vi "PID_set_ratio.vi"() -> ()   [LabVIEW 2016]
uses:
  <vilib>/addons/control/pid/autopid.llb/PID autotuning parameters (adv).ctl
  <vilib>/Analysis/baseanly.llb/Mean (DBL).vi
  <userlib>/Fluigent/Fluigent MFCS/FluigentMFCS_Full.llb/MFCS_EZ Detect.vi
  <userlib>/Fluigent/Fluigent MFCS/FluigentMFCS_Full.llb/MFCS_EZ Initialization.vi
  <userlib>/Fluigent/Fluigent MFCS/FluigentMFCS_Full.llb/MFCS_EZ Read All Channels Pressure.vi
  <userlib>/Fluigent/Fluigent MFCS/FluigentMFCS_Full.llb/MFCS_EZ Write Channel Pressure.vi
  <vilib>/addons/control/pid/NI_PID_autopid.lvlib
  <vilib>/Analysis/NI_AALBase.lvlib
  <vilib>/addons/control/pid/autopid.llb/PID Autotuning Design (Auto).vi
panel:
  out "F0 Stable":dbl=817.2839885789583 format="%0.2f"
  out "Fw Stable":dbl=490.71052053591 format="%0.2f"
  out "F1 Stable":dbl=326.5734680430485 format="%0.2f"
  in  "Stable?":bool=TRUE
  out "Measured Ratio":dbl[](graph)
  out "Flow Setpoint":dbl=326.3448275862069
  in  "Ratio Setpoint":dbl=0.4
  in  "Set PID Gains":T1={"proportional gain (Kc)"=0.5, "integral time (Ti, min)"=0.03, "derivative time (Td, min)"=0.0} {"derivative time (Td, min)" format="%#.6g"; "integral time (Ti, min)" format="%#.6g"; "proportional gain (Kc)" format="%#.6g"}
  in  "Channels":enum16{"1", "2", "3", "4", "5", "6", "7", "8"}[](array[ring])=[enum."5", enum."6", enum."8"]
  in  "Boards":enum16{"A", "B", "C"}[](array[ring])=[enum."A", enum."A", enum."A"]
  out "error out":errorcluster
  out "dt":dbl=0.023001670837402344
  in  "Filter Size":i32=5
  out "Filtered Flow":dbl=326.84827586206893 format="%0.2f"
  out "Feedback Signal":dbl[](graph)
  out "Current F1":dbl=325.82758620689657
  out "tuning completed?":bool
  in  "Accept new parameters":bool
  out "tuned PID gains":T1={"proportional gain (Kc)"=0.5, "integral time (Ti, min)"=0.03, "derivative time (Td, min)"=0.0} {"derivative time (Td, min)" format="%#.6g"; "integral time (Ti, min)" format="%#.6g"; "proportional gain (Kc)" format="%#.6g"}
  in  "auto? (F)":bool=TRUE
  in  "autotuning parameters":T2={"technique"=1, "type of controller"=1, "control specification"=0, "amplitude"=10.0} {"amplitude" format="%.2f"; "control specification" items=["normal", "fast", "slow"]; "type of controller" items=["P", "PI", "PID"]; "technique" items=["Step Open Loop", "Step Closed Loop", "Relay", "PID Relay"]}
  in  "reinitialize? (F)":bool=TRUE
  in  "autotune? (F)":bool
  in  "Manual Pressure Set":dbl=300.0
  in  "Feedback on":bool=TRUE
  out "Flow Rate":dbl[](graph)
  out "Pressure":dbl[](graph)
  in  "stop":bool
  out "Pressure":dbl=554.8080444335938
  out "Feedback Signal":dbl=-0.25172413793100645 format="%.2f"
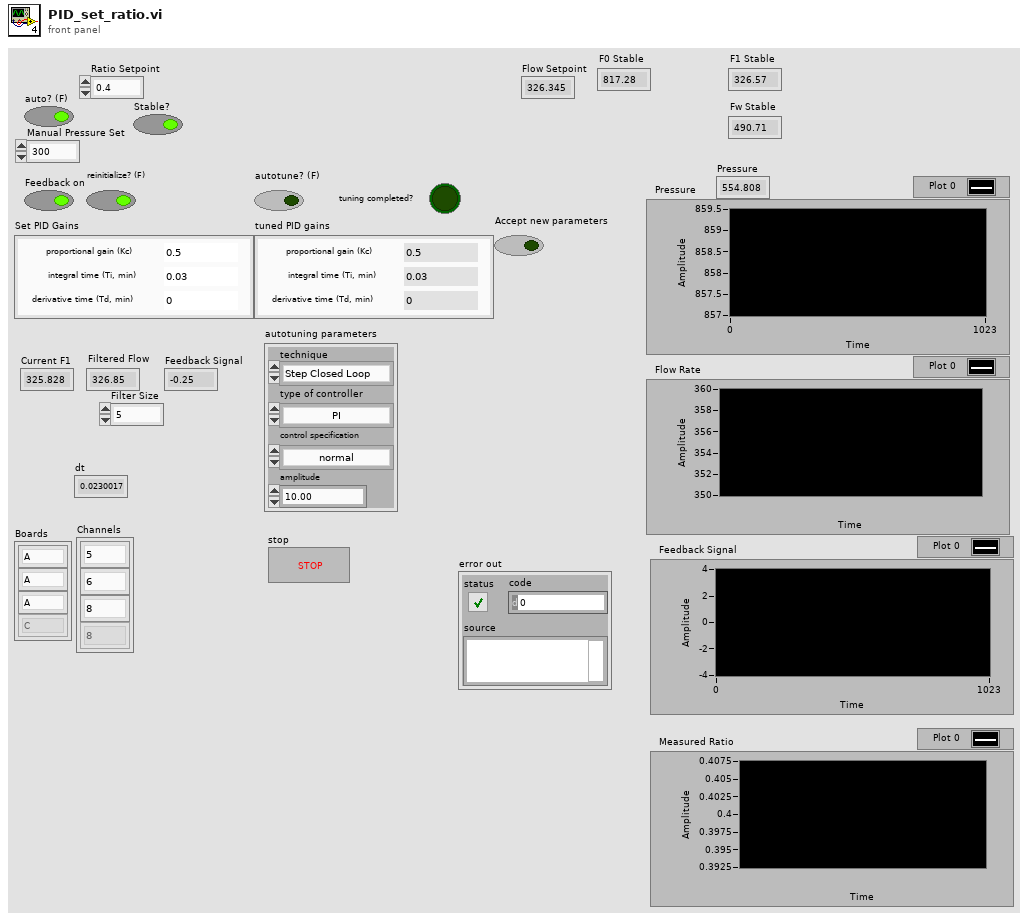
[diagram p1: front panel]
types:
  T1 = cluster{"proportional gain (Kc)":dbl, "integral time (Ti, min)":dbl, "derivative time (Td, min)":dbl}
  T2 = typedef "NI_PID_autopid.lvlib/PID autotuning parameters (adv).ctl" = cluster{"technique":u16, "type of controller":u16, "control specification":u16, "amplitude":dbl}
  T3 = typedef "_EZmfcsSN.ctl" = u16
  T4 = typedef "_frpRefNum" = refnum<k1>
  T5 = typedef "_EZmfcsRefNum.ctl" = refnum<k1>
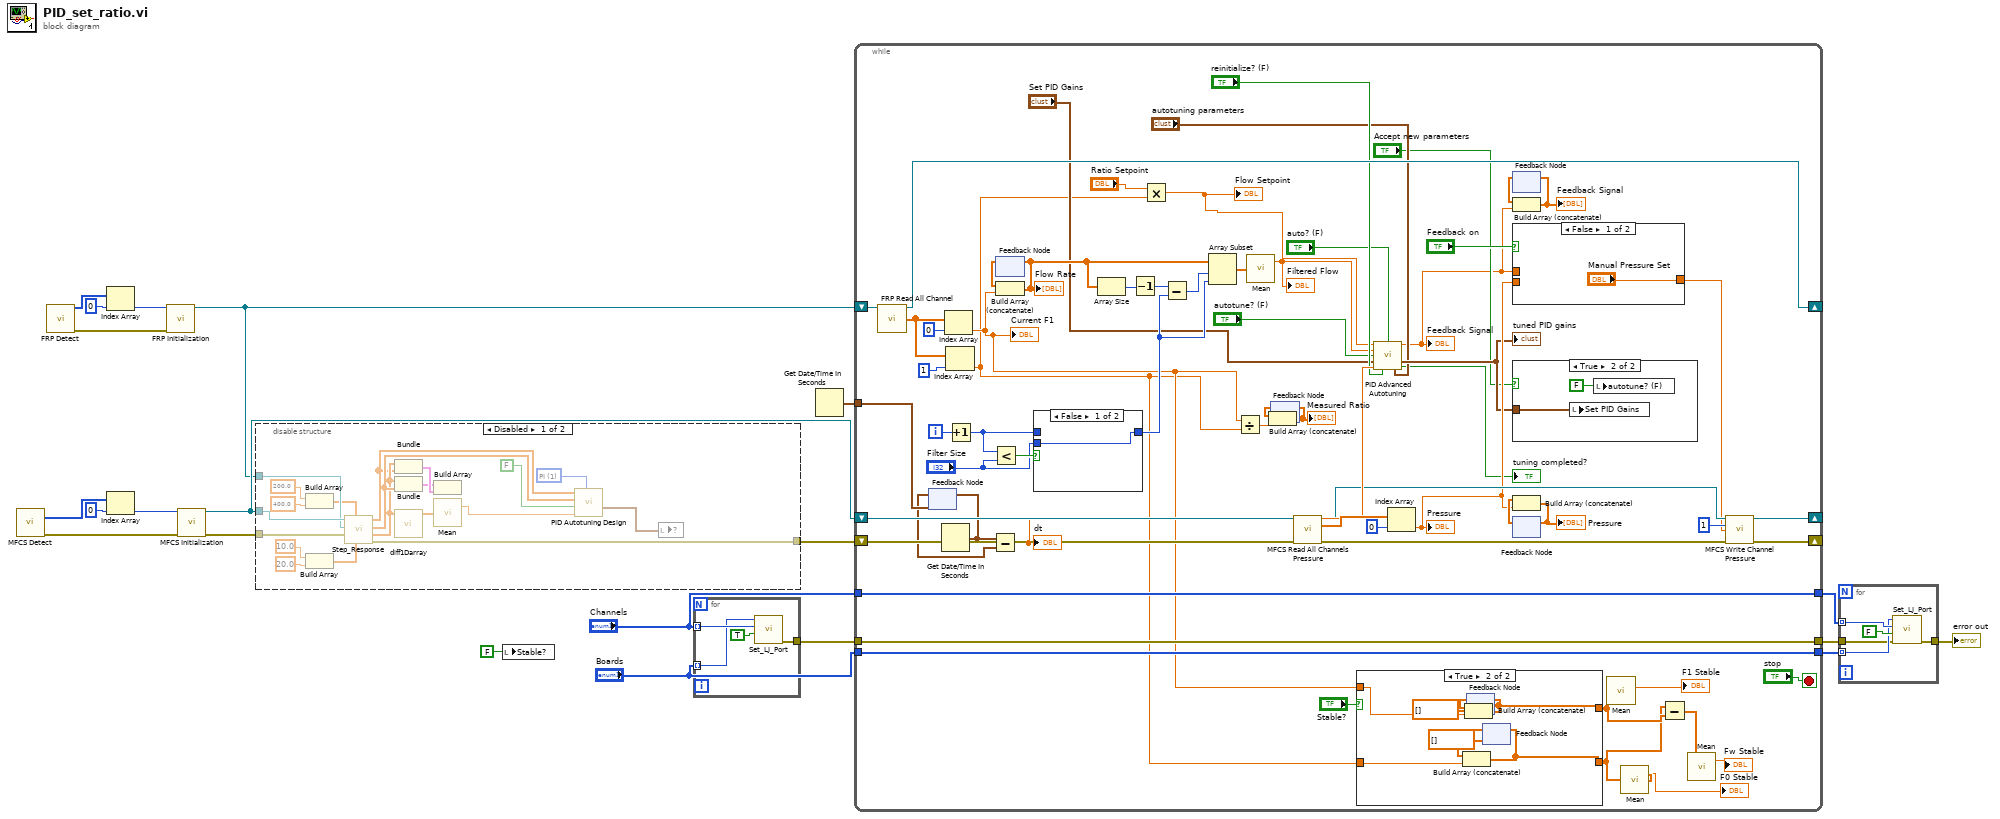
[diagram p0: block diagram]
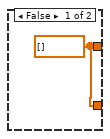
[diagram p3: hidden frame]
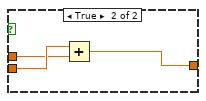
[diagram p6: hidden frame]
diagram:
  n1 = call-poly <userlib>:"MFCS Detect.vi"() -> ("[SN MFCS_EZ]"=w21:T3[], "error out"=w19:errorcluster)  [unwired: 14 in]
  n2 = call <userlib>:"FRP Detect.vi"() -> ("FLOWBOARD List"=w18:u16[], "error out"=w15:errorcluster)  [unwired: 14 in]
  n3 = Index Array(array=w18, index=0) -> (element=w14:u16)
  n4 = Index Array(array=w21, index=0) -> (element=w20:T3)
  n5 = call <userlib>:"FRP Initialization.vi"("Serial Number"=w14, "error in (no error)"=w15) -> ("FRP out"=w12:T4)  [unwired: 11 in, 2 out]
  n6 = call-poly <userlib>:"MFCS Initialization.vi"("SN MFCS_EZ"=w20, "error in (no error)"=w19) -> ("MFCS_EZ"=w13:T5, "error out"=w10:errorcluster)  [unwired: 11 in, 1 out]
  n7 = disable-structure shown="Disabled" {
    disable-tunnel: w13 -> [w43 _]
    disable-tunnel: w12 -> [w42 _]
    disable-tunnel: [w34 w44] -> w11
    disable-tunnel: w10 -> [w33 w44]
    frame Disabled {
      w38 = u16 1 items=["P", "PI", "PID"] ("Type of Controller")
      n8 = Build Array(200.0 ("element"), 400.0 ("element")) -> (w26:dbl[])
      n9 = Build Array(10.0 ("element"), 20.0 ("element")) -> (w27:dbl[])
      n10 = call "Step_Response.vi"("Times"=w27, "Pressure Sets"=w26, "MFCS Error"=w33, "FRP Handle"=w42, "MFCS Handle"=w43) -> ("error out"=w34:errorcluster, "T"=w25:dbl[], "Flow Rate"=w28:dbl[], "Pressure Setpoint"=w24:dbl[])  [unwired: 3 in]
      n11 = Bundle("T"=w25, "Pressure Setpoint"=w24) -> (w23:cluster{"T":dbl[], "Pressure Setpoint":dbl[]})  [unwired: 1 in]
      n12 = Bundle("T"=w25, "Flow Rate"=w28) -> (w22:cluster{"T":dbl[], "Flow Rate":dbl[]})  [unwired: 1 in]
      n13 = call "diff1Darray.vi"("Input"=w25) -> ("Diff"=w40:dbl[])  [unwired: 10 in]
      n14 = Build Array(w22, w23) -> ()  [unwired: 1 out]
      n15 = call-poly <vilib>:"Mean.vi"("X"=w40) -> ("mean"=w39:dbl)  [unwired: 1 out]
      n16 = call-poly <vilib>:"PID Autotuning Design.vi"("Type of Controller"=w38, "dt (s)"=w39, "closed-loop?"=FALSE, "Response signal"=w28, "Stimulus signal"=w24) -> ("PID gains"=w37:T1, "response operating point"=w35:dbl, "stimulus operating point"=w36:dbl)  [unwired: 3 in, 1 out]
      n17 = local write item#-1(w37) -> ()
    }
    frame Enabled {
    }
  }
  n18 = local write "Stable?"(FALSE ("Stable?")) -> ()
  n19 = for {
    tunnel: "Channels" -> [w48] mode=indexing
    tunnel: "Boards" -> [w47] mode=indexing
    tunnel: [w45] -> w8
    n20 = call "Set_LJ_Port.vi"("State"=TRUE, "Channel"=w48, "Flowboard"=w47) -> ("error out"=w45:errorcluster)  [unwired: 8 in]
  }
  n21 = Get Date/Time In Seconds() -> (seconds since 1Jan1904=w9:timestamp)
  n22 = while {
    shift-right: [w102] -> _
    shift-left: w11 -> [w111]
    shift-right: [w101] -> _
    shift-left: w13 -> [w112]
    shift-right: [w107] -> _
    shift-left: w12 -> [w108]
    tunnel: [w66] -> w3
    tunnel: w8 -> [w66]
    tunnel: w9 -> [w92]
    tunnel: "Boards" -> [w67]
    tunnel: "Channels" -> [w68]
    tunnel: [w68] -> w5
    tunnel: [w67] -> w4
    i -> [w79]
    stop <- "stop" stop-if-true
    n23 = call <userlib>:"FRP Read All Channel.vi"("FRP"=w108) -> ("FRP out"=w107:T4, "All Flow-Rates"=w64:dbl[])  [unwired: 12 in, 1 out]
    n24 = feedback #1(w92) -> (w90:timestamp)
    n25 = Get Date/Time In Seconds() -> (seconds since 1Jan1904=w91:timestamp)
    n26 = feedback-in #1(w91) -> ()
    n27 = Index Array(array=w64, index=0) -> (element=w56:dbl)
    "Current F1" <- w56
    n28 = Index Array(array=w64, index=1) -> (element=w55:dbl)
    n29 = Increment(x=w79) -> (x+1=w77:i32)
    n30 = Subtract(x=w91, y=w90) -> (x-y=w105:dbl)
    "dt" <- w105
    n31 = Less?(x=w77, y="Filter Size") -> (x < y?=w78:bool)
    n32 = feedback #2() -> (w96:dbl[])  [unwired: 1 in]
    n33 = Build Array (concatenate)(w96, w56) -> (w72:dbl[])
    "Flow Rate" <- w72
    n34 = feedback-in #2(w72) -> ()
    n35 = case shown="False" w78 {
      tunnel: w77 -> [_ w123]
      tunnel: [w122 w123] -> w74
      tunnel: "Filter Size" -> [w122 _]
      frame False {
      }
      frame True {
      }
    }
    n36 = Array Size(array=w72) -> (size(s)=w75:i32)
    n37 = Decrement(x=w75) -> (x-1=w73:i32)
    n38 = Multiply(x="Ratio Setpoint", y=w55) -> (x*y=w61:dbl)
    "Flow Setpoint" <- w61
    n39 = Subtract(x=w73, y=w74) -> (x-y=w71:i32)
    n40 = Array Subset(array=w72, index=w71, length=w74) -> (w70:dbl[])
    n41 = Divide(x=w56, y=w55) -> (x/y=w60:dbl)
    n42 = call-poly <vilib>:"Mean.vi"("X"=w70) -> ("mean"=w69:dbl)  [unwired: 1 out]
    "Filtered Flow" <- w69
    n43 = feedback #3() -> (w59:dbl[])  [unwired: 1 in]
    n44 = Build Array (concatenate)(w59, w60) -> (w58:dbl[])
    "Measured Ratio" <- w58
    n45 = feedback-in #3(w58) -> ()
    n46 = call-poly <userlib>:"MFCS Read All Channels Pressure.vi"("MFCS_EZ"=w112, "error in (no error)"=w111) -> ("MFCS_EZ out"=w104:T5, "All Channels Pressure"=w106:dbl[], "error out"=w103:errorcluster)  [unwired: 11 in]
    n47 = case shown="True" "Stable?" {
      tunnel: w56 -> [_ w121]
      tunnel: [w113 w119] -> w54
      tunnel: w55 -> [_ w117]
      tunnel: [w113 w116] -> w50
      frame False {
        w113 = dbl[] []
      }
      frame True {
        n48 = feedback #4(dbl[] []) -> (w120:dbl[])
        n49 = Build Array (concatenate)(w120, w121) -> (w119:dbl[])
        n50 = feedback-in #4(w119) -> ()
        n51 = feedback #5(dbl[] []) -> (w118:dbl[])
        n52 = Build Array (concatenate)(w118, w117) -> (w116:dbl[])
        n53 = feedback-in #5(w116) -> ()
      }
    }
    n54 = call <vilib>:"PID Advanced Autotuning.vi"("setpoint"=w61, "auto? (F)"="auto? (F)", "process variable"=w69, "autotune? (F)"="autotune? (F)", "PID gains"="Set PID Gains", "dt (s)"=w105, "reinitialize? (F)"="reinitialize? (F)", "autotuning parameters"="autotuning parameters") -> ("output"=w82:dbl, "tuned PID gains"=w88:T1, "tuning completed?"=→"tuning completed?":bool)  [unwired: 5 in]
    "Feedback Signal" <- w82
    "tuned PID gains" <- w88
    n55 = Index Array(array=w106, index=0) -> (element=w95:dbl)
    "Pressure" <- w95
    n56 = feedback #6() -> (w81:dbl[])  [unwired: 1 in]
    n57 = Build Array (concatenate)(w81, w82) -> (w80:dbl[])
    "Feedback Signal" <- w80
    n58 = feedback-in #6(w80) -> ()
    n59 = case shown="False" "Feedback on" {
      tunnel: w95 -> [_ w129]
      tunnel: w82 -> [_ w128]
      tunnel: ["Manual Pressure Set" w127] -> w94
      frame False {
      }
      frame True {
        n60 = Add(x=w129, y=w128) -> (x+y=w127:dbl)
      }
    }
    n61 = case shown="True" "Accept new parameters" {
      tunnel: w88 -> [_ w125]
      frame False {
      }
      frame True {
        n62 = local write "Set PID Gains"(w125) -> ()
        n63 = local write "autotune? (F)"(FALSE ("autotune? (F)")) -> ()
      }
    }
    n64 = feedback #7() -> (w98:dbl[])  [unwired: 1 in]
    n65 = Build Array (concatenate)(w98, w95) -> (w97:dbl[])
    "Pressure" <- w97
    n66 = feedback-in #7(w97) -> ()
    n67 = call-poly <vilib>:"Mean.vi"("X"=w54) -> ("mean"=→"F1 Stable":dbl)  [unwired: 1 out]
    n68 = call-poly <vilib>:"Mean.vi"("X"=w50) -> ("mean"=→"F0 Stable":dbl)  [unwired: 1 out]
    n69 = Subtract(x=w50, y=w54) -> (x-y=w52:dbl[])
    n70 = call-poly <vilib>:"Mean.vi"("X"=w52) -> ("mean"=→"Fw Stable":dbl)  [unwired: 1 out]
    n71 = call-poly <userlib>:"MFCS Write Channel Pressure.vi"("MFCS_EZ"=w104, "Channel Number (default=1)"=u8 1, "Pressure (mBar)"=w94, "error in (no error)"=w103) -> ("MFCS_EZ out"=w101:T5, "error out"=w102:errorcluster)  [unwired: 10 in]
  }
  n72 = for {
    tunnel: w5 -> [w134] mode=indexing
    tunnel: [w132] -> w2
    tunnel: w4 -> [w131] mode=indexing
    tunnel: w3 -> [w130]
    n73 = call "Set_LJ_Port.vi"("error in"=w130, "State"=FALSE, "Channel"=w134, "Flowboard"=w131) -> ("error out"=w132:errorcluster)  [unwired: 7 in]
  }
  "error out" <- w2
